vi "2photocell+ledcontrolv2.vi"() -> ()   [LabVIEW 2016]
uses:
  <vilib>/LabVIEW Interface for Arduino/LabVIEW Interface for Arduino.lvlib
  <vilib>/ptbypt/NI_PtbyPt.lvlib
panel:
  in  "Slide":dbl(slide) min=0.0 max=255.0 scale=0.0..255.0
  in  "Slide 2":dbl(slide) min=0.0 max=255.0 scale=0.0..255.0
  in  "Slide 3":dbl(slide) min=0.0 max=255.0 scale=0.0..255.0
  in  "Tab Control":enum32{"Page 1", "Page 2"}(tab)
  out "Voltage":dbl(knob) scale=0.0..5.0
  out "Filtered x":dbl format="%0.2f"
  out "Voltage 2":dbl(knob) scale=0.0..5.0
  out "Filtered x 2":dbl format="%0.2f"
  in  "br_coef":dbl
  in  "thrs low":i32=1
  in  "thrs high":i32=4
  in  "stop":bool
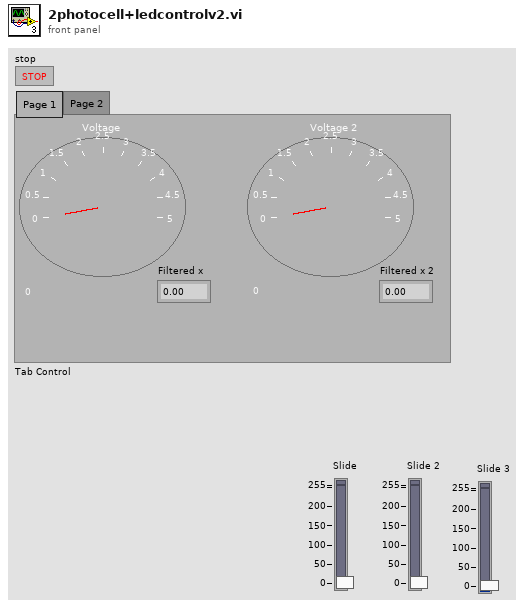
[diagram p1: front panel]
types:
  T1 = typedef "LabVIEW Interface for Arduino.lvlib/Arduino Resource.ctl" = cluster{"VISA resource":refnum<visa-resource-name>, "Board Type":T2, "Connection Type":enum8{"USB / Serial"}, "Bytes Per Packet (15)":u8}
  T2 = typedef "LabVIEW Interface for Arduino.lvlib/Board Type.ctl" = enum16{"Uno", "Dimuelanove w/Atmega 328", "Mega 2560"}
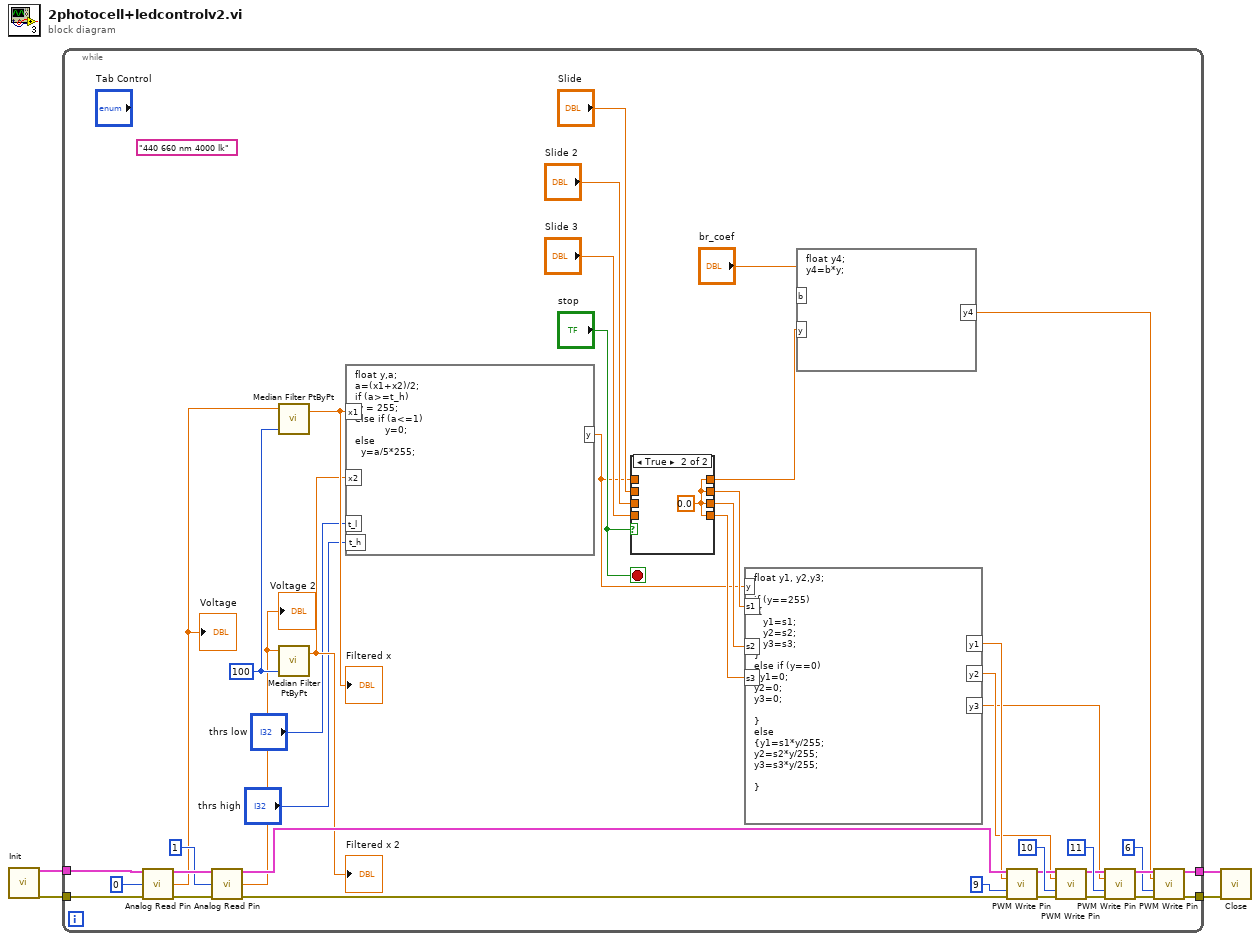
[diagram p0: block diagram]
diagram:
  n1 = call <vilib>:"Init.vi"() -> ("Arduino Resource"=w3:T1, "error out"=w4:errorcluster)  [unwired: 18 in]
  n2 = while {
    tunnel: w4 -> [w42]
    tunnel: w3 -> [w37]
    tunnel: [w12] -> w2
    tunnel: [w11] -> w1
    stop <- "stop" stop-if-true
    (unwired) "440 660 nm 4000 lk"
    w35 = 100 ("rank")
    n3 = call <vilib>:"Analog Read Pin.vi"("Arduino Resource"=w37, "Analog Input Pin (0)"=u8 0, "error in"=w42) -> ("Arduino Resource"=w45:T1, "Voltage"=w36:dbl, "error out"=w41:errorcluster)  [unwired: 10 in]
    "Voltage" <- w36
    n4 = call <vilib>:"Analog Read Pin.vi"("Arduino Resource"=w45, "Analog Input Pin (0)"=u8 1, "error in"=w41) -> ("Arduino Resource"=w40:T1, "Voltage"=w34:dbl, "error out"=w39:errorcluster)  [unwired: 10 in]
    "Voltage 2" <- w34
    n5 = call <vilib>:"Median Filter PtByPt.vi"("rank"=w35, "x"=w36) -> ("Filtered x"=w33:dbl)  [unwired: 2 in, 1 out]
    "Filtered x" <- w33
    n6 = call <vilib>:"Median Filter PtByPt.vi"("rank"=w35, "x"=w34) -> ("Filtered x"=w32:dbl)  [unwired: 2 in, 1 out]
    "Filtered x 2" <- w32
    n7 = formula code="float y,a;\na=(x1+x2)/2;\nif (a>=t_h)\n y = 255;\nelse if (a<=1)\n          y=0;\nelse\n  y=a/5*255;"("x1"=w33, "x2"=w32, "t_l"="thrs low", "t_h"="thrs high") -> ("y"=w8:dbl)
    n8 = case shown="True" "stop" {
      tunnel: "Slide 2" -> [w49 _]
      tunnel: [w49 w50] -> w18
      tunnel: "Slide 3" -> [w48 _]
      tunnel: [w48 w50] -> w17
      tunnel: "Slide" -> [w47 _]
      tunnel: [w47 w50] -> w19
      tunnel: w8 -> [w46 _]
      tunnel: [w46 w50] -> w6
      frame False {
      }
      frame True {
        w50 = 0.0 ("Slide 2")
      }
    }
    n9 = formula code="float y1, y2,y3;\n\nif (y==255)\n {\n   y1=s1;\n   y2=s2;\n   y3=s3;\n}\nelse if (y==0)\n{y1=0;\ny2=0;\ny3=0;\n\n}\nelse \n{y1=s1*y/255;\ny2=s2*y/255;\ny3=s3*y/255;\n\n}"("s1"=w19, "s2"=w18, "s3"=w17, "y"=w8) -> ("y1"=w16:dbl, "y2"=w15:dbl, "y3"=w14:dbl)
    n10 = formula code="float y4;\ny4=b*y;"("b"="br_coef", "y"=w6) -> ("y4"=w5:dbl)
    n11 = call <vilib>:"PWM Write Pin.vi"("Arduino Resource"=w40, "Duty Cycle (0 - 255)"=w16, "PWM Pin (3)"=u8 9, "error in"=w39) -> ("Arduino Resource"=w25:T1, "error out"=w21:errorcluster)  [unwired: 10 in]
    n12 = call <vilib>:"PWM Write Pin.vi"("Arduino Resource"=w25, "Duty Cycle (0 - 255)"=w15, "PWM Pin (3)"=u8 10, "error in"=w21) -> ("Arduino Resource"=w24:T1, "error out"=w20:errorcluster)  [unwired: 10 in]
    n13 = call <vilib>:"PWM Write Pin.vi"("Arduino Resource"=w24, "Duty Cycle (0 - 255)"=w14, "PWM Pin (3)"=u8 11, "error in"=w20) -> ("Arduino Resource"=w13:T1, "error out"=w10:errorcluster)  [unwired: 10 in]
    n14 = call <vilib>:"PWM Write Pin.vi"("Arduino Resource"=w13, "Duty Cycle (0 - 255)"=w5, "PWM Pin (3)"=u8 6, "error in"=w10) -> ("Arduino Resource"=w12:T1, "error out"=w11:errorcluster)  [unwired: 10 in]
  }
  n15 = call <vilib>:"Close.vi"("Arduino Resource"=w2, "error in"=w1) -> ()  [unwired: 13 in, 1 out]
